vi "Sets the ARC mode status for MANU.vi"(5 "Enable to Query the ARC mode":bool, 7 "Enable to Setup the ARC mode":bool, 8 "error in":errorcluster, 10 "ARC mode":u8(ring) items=["OFF", "ON_CONT", "ON_STOP"], 11 "VISA resource name":refnum<visa-resource-name>) -> (0 "error out":errorcluster, 2 "Return the ARC mode":string, 3 "VISA resource name out":refnum<visa-resource-name>)   [LabVIEW 2011, in "GPT-9000.lvlib"]
uses:
  <instrlib>/GPT-9000/GPT-9000.lvlib
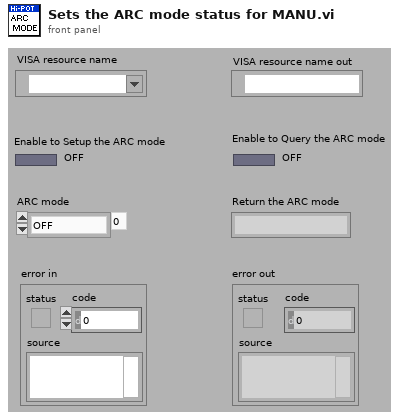
[diagram p1: front panel]
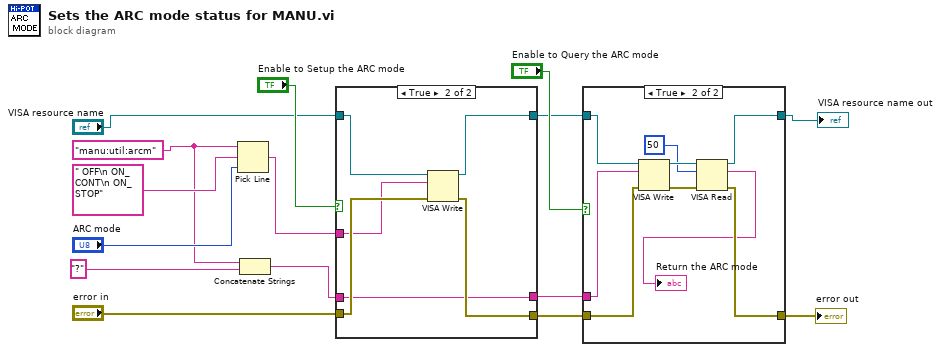
[diagram p0: block diagram]
diagram:
  w12 = "manu:util:arcm"
  n1 = Pick Line(string ("")=w12, multi-line string=" OFF\n ON_CONT\n ON_STOP", line index="ARC mode") -> (output string=w10:string)
  n2 = Concatenate Strings(w12, "?") -> (w9:string)
  n3 = case shown="True" "Enable to Setup the ARC mode" {
    tunnel: w10 -> [_ w19]
    tunnel: w9 -> [w16 w20]
    tunnel: "VISA resource name" -> [w18 w24]
    tunnel: "error in" -> [w17 w23]
    tunnel: [w18 w22] -> w5
    tunnel: [w17 w21] -> w4
    tunnel: [w16 w20] -> w3
    frame False {
    }
    frame True {
      n4 = VISA Write(VISA resource name=w24, write buffer=w19, error in (no error)=w23) -> (VISA resource name out=w22:refnum<visa-resource-name>, error out=w21:errorcluster)  [unwired: 1 out]
    }
  }
  n5 = case shown="True" "Enable to Query the ARC mode" {
    tunnel: w5 -> [w26 w32]
    tunnel: w4 -> [w25 w31]
    tunnel: w3 -> [_ w30]
    tunnel: [w26 w29] -> w2
    tunnel: [w25 w28] -> w1
    frame False {
    }
    frame True {
      n6 = VISA Write(VISA resource name=w32, write buffer=w30, error in (no error)=w31) -> (VISA resource name out=w34:refnum<visa-resource-name>, error out=w35:errorcluster)  [unwired: 1 out]
      n7 = VISA Read(VISA resource name=w34, byte count=u32 50, error in (no error)=w35) -> (VISA resource name out=w29:refnum<visa-resource-name>, read buffer=→"Return the ARC mode":string, error out=w28:errorcluster)  [unwired: 1 out]
    }
  }
  "VISA resource name out" <- w2
  "error out" <- w1
